vi "NI 9775 Getting Started Record Mode (FPGA).vi"() -> ()   [LabVIEW 2021]
uses:
  <vilib>/LabVIEW Targets/FPGA/cRIO/shared/nicrio_ModuleControls/nicrio_BasicConversionTime.ctl
  <vilib>/LabVIEW Targets/FPGA/cRIO/shared/nicrio_ModuleControls/nicrio_cRIO-9775_RecordDataRates4ChansRing.ctl
  <vilib>/LabVIEW Targets/FPGA/cRIO/shared/nicrio_ModuleControls/nicrio_cRIO-9775_TriggerConfigCal.ctl
  <vilib>/LabVIEW Targets/FPGA/cRIO/shared/nicrio_ModuleControls/nicrio_cRIO-9775_TriggerSlope.ctl
  <vilib>/rvi/eio/common/nirviEmuTemplatePropertySet_errors.vi
  <vilib>/rvi/eio/common/nirviEmuTemplateMethod_errors.vi
  <vilib>/rvi/Emulation/niFpgaGetClockAttributes.vi
  <vilib>/rvi/Emulation/niFpgaSctlEmulationGetInTimedLoop.vi
  <vilib>/rvi/Emulation/niFpgaEmulationReportErrorSimple.vi
  <vilib>/rvi/interface/RandomDataEmulation/niFpgaRandomDataHandleErrors.vi
  <vilib>/rvi/Emulation/niFpgaCriticalErrorInLSC.vi
  <vilib>/eio/EIOPropertyNode/EIOPropertyNode.xnode
  <vilib>/eio/EIONode/EIONode.xnode
  <vilib>/eio/EIOMethodNode/EIOMethodNode.xnode
  <vilib>/rvi/DataTransferAndStorage/Container/XNode/niFpgaContainer.xnode
  <vilib>/rvi/interface/RandomDataEmulation/nirviRandomDataFpgaReadWriteTemplate.vi
  <vilib>/rvi/eio/common/nirviEmuTemplatePropertyGet_errors.vi
  <vilib>/rvi/eio/common/nirviEmuTemplatePropertyGet_noerrors.vi
  <vilib>/rvi/eio/common/nirviEmuTemplatePropertySet_noerrors.vi
panel:
  in  "Trigger Record Timeout (Ticks)":i32
  in  "PreTrigger Samples per Record":u32
  in  "Samples per Record":u32
  in  "Trigger Type":T1(tab)
  in  "AI Trigger Configuration":T3
  in  "AI 0 Trigger Configuration":T4
  in  "AI 1 Trigger Configuration":T4
  in  "AI 2 Trigger Configuration":T4
  in  "AI 3 Trigger Configuration":T4
  in  "Enable Low Pass Filter":T5
  out "FPGA Error Out":errorcluster
  out "Fetch Timed Out":bool
  in  "Fetch Timeout (Ticks)":i32
  out "Trigger Record Timed Out":bool
  in  "Record Data Rate":T6=1 items=["20.000 MS/s (NI 9775)"=1, "10.00 MS/s (NI 9775)"=2, "6.667 MS/s (NI 9775)"=3, "5.000 MS/s (NI 9775)"=4, "2.500 MS/s (NI 9775)"=8, "1.667 MS/s (NI 9775)"=12, "1.250 MS/s (NI 9775)"=16, "1.000 MS/s (NI 9775)"=20, "833.333 KS/s (NI 9775)"=24, "714.286 KS/s (NI 9775)"=28, "625.000 KS/s (NI 9775)"=32, "555.556 KS/s (NI 9775)"=36, "500.000 KS/s (NI 9775)"=40, "454.545 KS/s (NI 9775)"=44, "416.667 KS/s (NI 9775)"=48, "384.615 KS/s (NI 9775)"=52, "357.143 KS/s (NI 9775)"=56, "333.333 KS/s (NI 9775)"=60, "312.500 KS/s (NI 9775)"=64, "294.118 KS/s (NI 9775)"=68, "277.778 KS/s (NI 9775)"=72, "263.158 KS/s (NI 9775)"=76, "250.000 KS/s (NI 9775)"=80, "238.095 KS/s (NI 9775)"=84, "227.273 KS/s (NI 9775)"=88, "217.391 KS/s (NI 9775)"=92, "208.333 KS/s (NI 9775)"=96, "200.000 KS/s (NI 9775)"=100, "192.308 KS/s (NI 9775)"=104, "185.185 KS/s (NI 9775)"=108, "178.571 KS/s (NI 9775)"=112, "172.414 KS/s (NI 9775)"=116, "166.667 KS/s (NI 9775)"=120, "161.290 KS/s (NI 9775)"=124, "156.250 KS/s (NI 9775)"=128, "151.515 KS/s (NI 9775)"=132, "147.059 KS/s (NI 9775)"=136, "142.857 KS/s (NI 9775)"=140, "138.889 KS/s (NI 9775)"=144, "135.135 KS/s (NI 9775)"=148, "131.579 KS/s (NI 9775)"=152, "128.205 KS/s (NI 9775)"=156, "125.000 KS/s (NI 9775)"=160, "121.951 KS/s (NI 9775)"=164, "119.048 KS/s (NI 9775)"=168, "116.279 KS/s (NI 9775)"=172, "113.636 KS/s (NI 9775)"=176, "111.111 KS/s (NI 9775)"=180, "108.696 KS/s (NI 9775)"=184, "106.383 KS/s (NI 9775)"=188, "104.167 KS/s (NI 9775)"=192, "102.041 KS/s (NI 9775)"=196, "100.000 KS/s (NI 9775)"=200, "50.000 KS/s (NI 9775)"=400, "33.333 KS/s (NI 9775)"=600, "25.000 KS/s (NI 9775)"=800, "20.000 KS/s (NI 9775)"=1000, "16.667 KS/s (NI 9775)"=1200, "14.286 KS/s (NI 9775)"=1400, "12.500 KS/s (NI 9775)"=1600, "11.111 KS/s (NI 9775)"=1800, "10.000 KS/s (NI 9775)"=2000, "9.091 KS/s (NI 9775)"=2200, "8.333 KS/s (NI 9775)"=2400, "7.692 KS/s (NI 9775)"=2600, "7.143 KS/s (NI 9775)"=2800, "6.667 KS/s (NI 9775)"=3000, "6.250 KS/s (NI 9775)"=3200, "5.882 KS/s (NI 9775)"=3400, "5.556 KS/s (NI 9775)"=3600, "5.000 KS/s (NI 9775)"=4000, "4.762 KS/s (NI 9775)"=4200, "4.545 KS/s (NI 9775)"=4400, "4.348 KS/s (NI 9775)"=4600, "4.167 KS/s (NI 9775)"=4800, "4.000 KS/s (NI 9775)"=5000, "3.846 KS/s (NI 9775)"=5200, "3.571 KS/s (NI 9775)"=5600, "3.333 KS/s (NI 9775)"=6000, "3.125 KS/s (NI 9775)"=6400, "2.941 KS/s (NI 9775)"=6800, "2.778 KS/s (NI 9775)"=7200, "2.632 KS/s (NI 9775)"=7600, "2.500 KS/s (NI 9775)"=8000, "2.381 KS/s (NI 9775)"=8400, "2.273 KS/s (NI 9775)"=8800, "2.174 KS/s (NI 9775)"=9200, "2.083 KS/s (NI 9775)"=9600, "2.000 KS/s (NI 9775)"=10000, "1.923 KS/s (NI 9775)"=10400, "1.852 KS/s (NI 9775)"=10800, "1.786 KS/s (NI 9775)"=11200, "1.724 KS/s (NI 9775)"=11600, "1.667 KS/s (NI 9775)"=12000, "1.613 KS/s (NI 9775)"=12400, "1.563 KS/s (NI 9775)"=12800, "1.515 KS/s (NI 9775)"=13200, "1.471 KS/s (NI 9775)"=13600, "1.429 KS/s (NI 9775)"=14000, "1.389 KS/s (NI 9775)"=14400, "1.351 KS/s (NI 9775)"=14800, "1.316 KS/s (NI 9775)"=15200, "1.282 KS/s (NI 9775)"=15600, "1.250 KS/s (NI 9775)"=16000, "1.220 KS/s (NI 9775)"=16400, "1.190 KS/s (NI 9775)"=16800, "1.163 KS/s (NI 9775)"=17200, "1.136 KS/s (NI 9775)"=17600, "1.111 KS/s (NI 9775)"=18000, "1.087 KS/s (NI 9775)"=18400, "1.064 KS/s (NI 9775)"=18800, "1.042 KS/s (NI 9775)"=19200, "1.020 KS/s (NI 9775)"=19600, "1.000 KS/s (NI 9775)"=20000, "0.980 KS/s (NI 9775)"=20400, "0.962 KS/s (NI 9775)"=20800, "0.943 KS/s (NI 9775)"=21200, "0.926 KS/s (NI 9775)"=21600, "0.909 KS/s (NI 9775)"=22000, "0.893 KS/s (NI 9775)"=22400, "0.877 KS/s (NI 9775)"=22800, "0.862 KS/s (NI 9775)"=23200, "0.847 KS/s (NI 9775)"=23600, "0.833 KS/s (NI 9775)"=24000, "0.820 KS/s (NI 9775)"=24400, "0.806 KS/s (NI 9775)"=24800, "0.794 KS/s (NI 9775)"=25200, "0.781 KS/s (NI 9775)"=25600, "0.694 KS/s (NI 9775)"=28800, "0.625 KS/s (NI 9775)"=32000, "0.568 KS/s (NI 9775)"=35200, "0.521 KS/s (NI 9775)"=38400, "0.446 KS/s (NI 9775)"=44800, "0.391 KS/s (NI 9775)"=51200, "0.347 KS/s (NI 9775)"=57600, "0.313 KS/s (NI 9775)"=64000]
  in  "Timing Mode":T7
  # "Overview: Demonstrates how to acquire record (triggered) data from the NI 9775\nRequirements: LabVIEW Full Development System, LV FPGA, and NI RIO\nInstructions: \n1. Run NI 9775 Getting Started Record Mode (Host).vi"
  # "Output Parameters"
  # "Timing Parameters"
  # "Input Parameters"
  # "Trigger Parameters"
  # "This tab is intentionally left blank. The FPGA will automatically trigger the NI 9775."
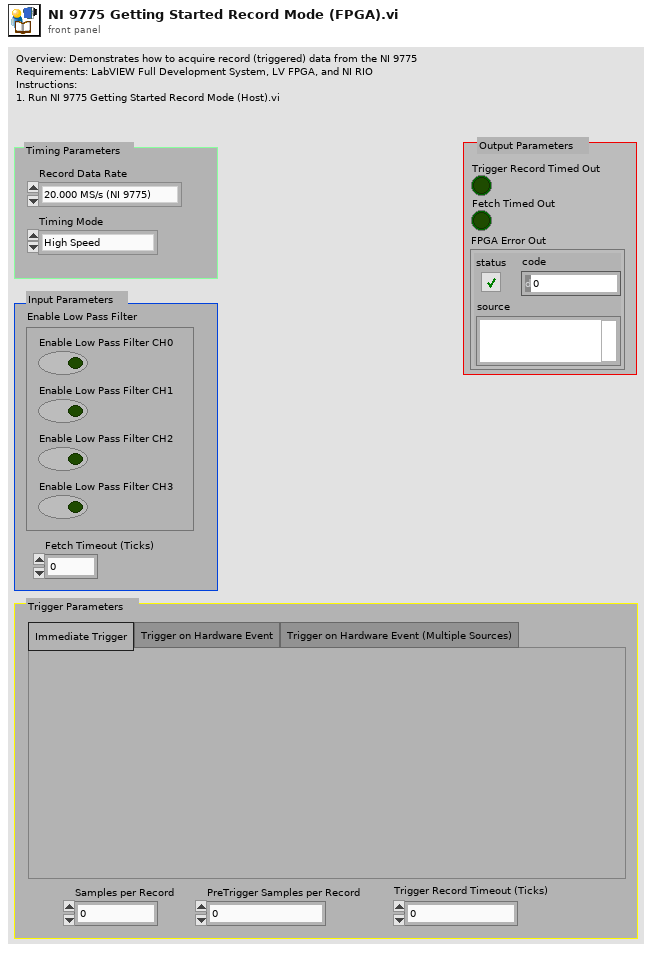
[diagram p1: front panel]
types:
  T1 = enum32{"Immediate Trigger", "Trigger on Hardware Event", "Trigger on Hardware Event (Multiple Sources)"}
  T2 = typedef "nicrio_cRIO-9775_TriggerSlope.ctl" = enum8{"Positive", "Negative"}
  T3 = cluster{"Trigger Slope":T2, "Trigger Level":fxp<+/-,17,5>, "Hystesis Value":fxp<+,16,4>, "AI Channel":u8}
  T4 = typedef "nicrio_cRIO-9775_TriggerConfigCal.ctl" = cluster{"Enable":bool, "Trigger Slope":T2, "Trigger Level":fxp<+/-,17,5>, "Hystesis Value":fxp<+,16,4>}
  T5 = cluster{"Enable Low Pass Filter CH1":bool, "Enable Low Pass Filter CH2":bool, "Enable Low Pass Filter CH3":bool, "Enable Low Pass Filter CH0":bool}
  T6 = typedef "nicrio_cRIO-9775_RecordDataRates4ChansRing.ctl" = u16
  T7 = typedef "nicrio_BasicConversionTime.ctl" = enum8{"High Speed", "High Resolution"}
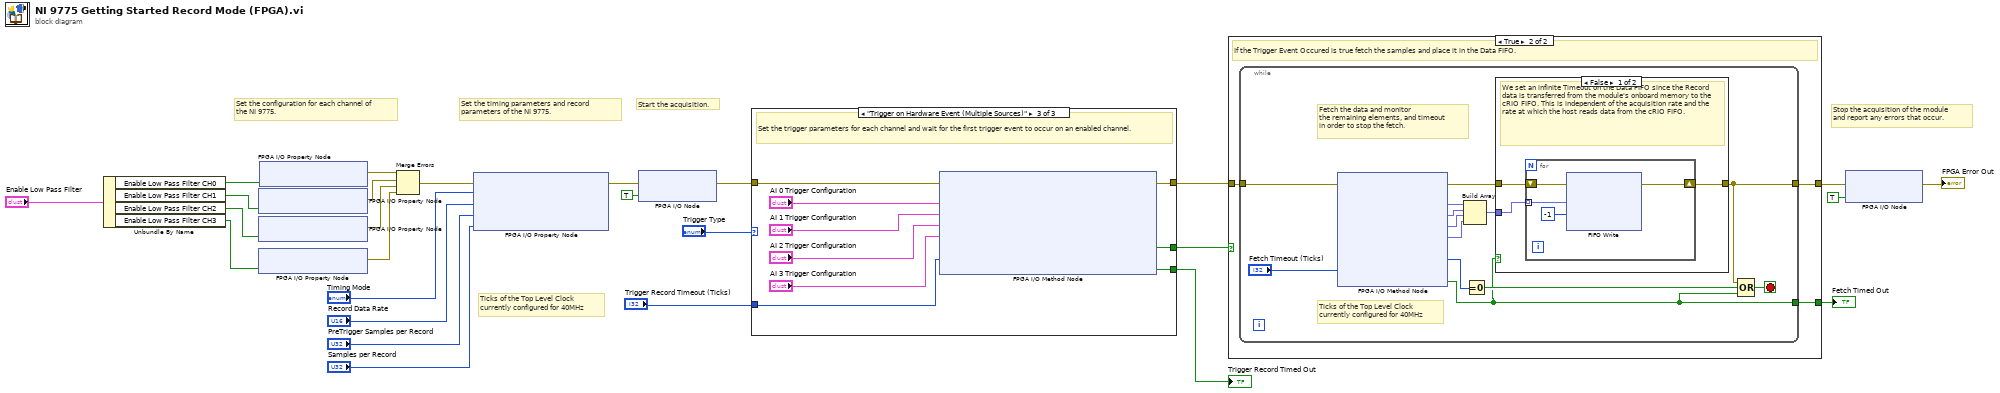
[diagram p0: block diagram]
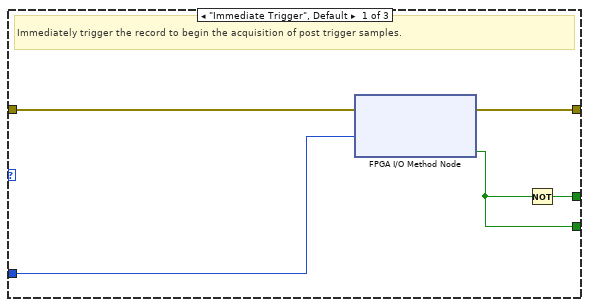
[diagram p2: hidden frame]
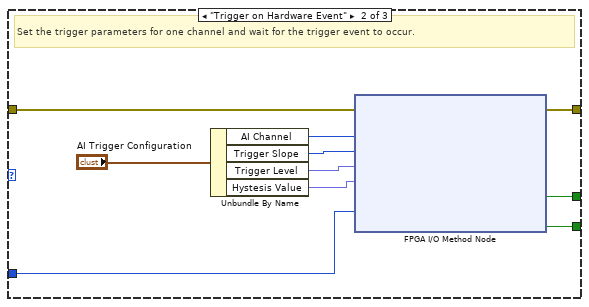
[diagram p3: hidden frame]
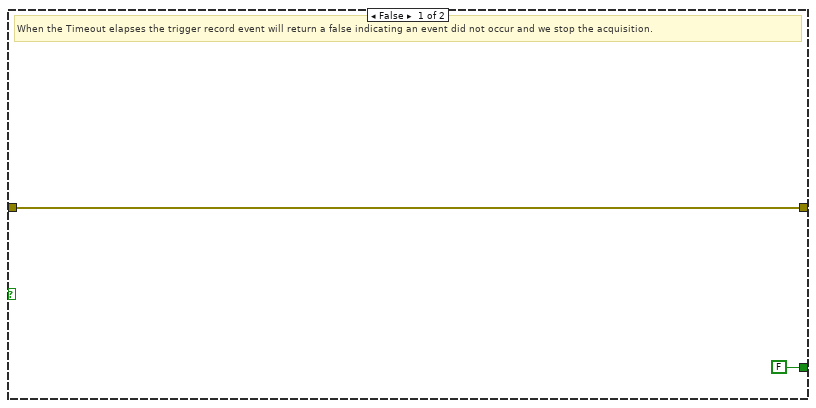
[diagram p4: hidden frame]
diagram:
  # "Ticks of the Top Level Clock\ncurrently configured for 40MHz"
  # "Stop the acquisition of the module \nand report any errors that occur."
  # "Start the acquisition."
  # "Set the timing parameters and record parameters of the NI 9775."
  # "Set the configuration for each channel of the NI 9775."
  n1 = Unbundle By Name("Enable Low Pass Filter") -> ("Enable Low Pass Filter CH0"=w5:bool, "Enable Low Pass Filter CH1"=w4:bool, "Enable Low Pass Filter CH2"=w3:bool, "Enable Low Pass Filter CH3"=w2:bool)
  n2 = xnode "FPGA I/O Property Node"("Enable Analog Filter"=w4) -> ("error out"=w21:errorcluster)  [unwired: 2 in, 1 out]
  n3 = xnode "FPGA I/O Property Node"("Enable Analog Filter"=w3) -> ("error out"=w20:errorcluster)  [unwired: 2 in, 1 out]
  n4 = xnode "FPGA I/O Property Node"("Enable Analog Filter"=w2) -> ("error out"=w19:errorcluster)  [unwired: 2 in, 1 out]
  n5 = xnode "FPGA I/O Property Node"("Enable Analog Filter"=w5) -> ("error out"=w23:errorcluster)  [unwired: 2 in, 1 out]
  n6 = Merge Errors(w23, w21, w20, w19) -> (w22:errorcluster)
  n7 = xnode "FPGA I/O Property Node"("error in"=w22, "Timing Mode"="Timing Mode", "Record Data Rate"="Record Data Rate", "Record PreTrigger Samples"="PreTrigger Samples per Record", "Record Samples"="Samples per Record") -> ("error out"=w13:errorcluster)  [unwired: 1 in, 1 out]
  n8 = xnode "FPGA I/O Node"("error in"=w13, "Mod1/Start"=TRUE) -> ("error out"=w11:errorcluster)  [unwired: 1 in, 1 out]
  n9 = case shown="\"Trigger on Hardware Event (Multiple Sources)\"" "Trigger Type" {
    tunnel: w11 -> [w30 w40 w50]
    tunnel: [w31 w41 w49] -> w10
    tunnel: [w29 w38 w48] -> w9
    tunnel: [w27 w37 w47] -> w8
    tunnel: "Trigger Record Timeout (Ticks)" -> [w28 w39 w45]
    frame "Immediate Trigger", Default {
      # "Immediately trigger the record to begin the acquisition of post trigger samples."
      n10 = xnode "FPGA I/O Method Node"("error in"=w30, "Timeout (Ticks)"=w28) -> ("error out"=w31:errorcluster, "Timed Out"=w29:bool)  [unwired: 1 in, 1 out]
      n11 = Not(x=w29) -> (.not. x?=w27:bool)
    }
    frame "Trigger on Hardware Event" {
      # "Set the trigger parameters for one channel and wait for the trigger event to occur."
      n12 = Unbundle By Name("AI Trigger Configuration") -> ("AI Channel"=w35:u8, "Trigger Slope"=w34:T2, "Trigger Level"=w33:fxp<+/-,17,5>, "Hystesis Value"=w32:fxp<+,16,4>)
      n13 = xnode "FPGA I/O Method Node"("error in"=w40, "AI Channel"=w35, "Trigger Slope"=w34, "Trigger Level"=w33, "Hysteresis Value"=w32, "Timeout (Ticks)"=w39) -> ("error out"=w41:errorcluster, "Trigger Event Occurred"=w37:bool, "Timed Out"=w38:bool)  [unwired: 1 in, 1 out]
    }
    frame "Trigger on Hardware Event (Multiple Sources)" {
      # "Set the trigger parameters for each channel and wait for the first trigger event to occur on an enabled channel."
      n14 = xnode "FPGA I/O Method Node"("error in"=w50, "AI 0 Trigger Configuration"="AI 0 Trigger Configuration", "AI 1 Trigger Configuration"="AI 1 Trigger Configuration", "AI 2 Trigger Configuration"="AI 2 Trigger Configuration", "AI 3 Trigger Configuration"="AI 3 Trigger Configuration", "Timeout (Ticks)"=w45) -> ("error out"=w49:errorcluster, "Trigger Event Occurred"=w47:bool, "Timed Out"=w48:bool)  [unwired: 1 in, 1 out]
    }
  }
  "Trigger Record Timed Out" <- w9
  n15 = case shown="True" w8 {
    tunnel: [w51 w55] -> w26
    tunnel: [FALSE ("Timed Out") w53] -> w14
    tunnel: w10 -> [w51 w54]
    frame False {
      # "When the Timeout elapses the trigger record event will return a false indicating an event did not occur and we stop the acquisition."
    }
    frame True {
      # "If the Trigger Event Occured is true fetch the samples and place it in the Data FIFO."
      n16 = while {
        tunnel: [w66] -> w55
        tunnel: w54 -> [w65]
        tunnel: [w56] -> w53
        stop <- w67 stop-if-true
        # "Ticks of the Top Level Clock\ncurrently configured for 40MHz"
        # "Fetch the data and monitor\nthe remaining elements, and timeout \nin order to stop the fetch."
        n17 = xnode "FPGA I/O Method Node"("error in"=w65, "Timeout (Ticks)"="Fetch Timeout (Ticks)") -> ("error out"=w64:errorcluster, "AI0"=w62:fxp<+/-,17,5>, "AI1"=w61:fxp<+/-,17,5>, "AI2"=w60:fxp<+/-,17,5>, "AI3"=w59:fxp<+/-,17,5>, "Elements Remaining"=w58:u32, "Timed Out"=w56:bool)  [unwired: 1 in, 2 out]
        n18 = Build Array(w62, w61, w60, w59) -> (w68:fxp<+/-,17,5>[])
        n19 = Equal To 0?(x=w58) -> (x = 0?=w57:bool)
        n20 = case shown="False" w56 {
          tunnel: w68 -> [w71 _]
          tunnel: [w70 w76] -> w66
          tunnel: w64 -> [w69 w76]
          frame False {
            # "We set an infinite Timeout on the Data FIFO since the Record data is transferred from the module's onboard memory to the cRIO FIFO. This is independent of the acquisition rate and the rate at which the host reads data from the cRIO FIFO."
            n21 = for {
              tunnel: w71 -> [w72] mode=indexing
              shift-right: [w74] -> w70
              shift-left: w69 -> [w73]
              n22 = xnode ("FIFO Write")("Element"=w72, "Timeout"=-1 ("Timeout (-1 for no timeout)"), "error in (no error)"=w73) -> ("error out"=w74:errorcluster)  [unwired: 1 in, 2 out]
            }
          }
          frame True {
            # "If the fetch times out we prevent data from being entered into the FIFO"
          }
        }
        n23 = Compound Arithmetic op=OR(w66, w57, w56) -> (w67:bool)
      }
    }
  }
  "Fetch Timed Out" <- w14
  n24 = xnode "FPGA I/O Node"("error in"=w26, "Mod1/Stop"=TRUE) -> ("error out"=→"FPGA Error Out":errorcluster)  [unwired: 1 in, 1 out]
